vi "Lookup Message Channels.vi"(8 "error in (no error)":errorcluster, 10 "Message Channels in":T3 {"Status" format="%.0x"; "Triggers" format="%.0x"; "Periodic Enable" format="%.0x"}, 11 "Section Ref in":T2 format="%.0x") -> (0 "error out":errorcluster, 1 "Trigger Parameters":T1, 2 "Message Channels out":T3 {"Status" format="%.0x"; "Triggers" format="%.0x"; "Periodic Enable" format="%.0x"}, 3 "Section Ref out":T2 format="%.0x")   [LabVIEW 2015, in "Instrument Addon System Explorer.lvlib"]
uses:
  Instrument Addon System Explorer.lvlib
  Types/Message Channel Lookup Cluster.ctl
  <vilib>/NI Veristand/Custom Device API/Custom Device Item Ref.ctl
  Shared/Types/Trigger Parameters.ctl
  Shared/Types/FG Control.ctl
  <vilib>/NI Veristand/Custom Device Tools/Custom Device Utility Library/NI VeriStand - Search for Item by GUID.vi
  <vilib>/NI Veristand/Custom Device API/NI VeriStand - Set Item Property.vi
  <vilib>/NI Veristand/Custom Device API/Set Item Property (String).vi
  <vilib>/NI Veristand/Custom Device API/Set Item Property (Boolean).vi
  <vilib>/NI Veristand/Custom Device API/NI VeriStand - Get Item Property.vi
  <vilib>/NI Veristand/Custom Device API/Get Item Property (String).vi
  <vilib>/NI Veristand/Custom Device API/Get Item Property (Boolean).vi
  Shared/Constants.vi
  <vilib>/NI Veristand/Custom Device Tools/Custom Device Utility Library/Custom Device Utility Library.lvlib
  Shared/Instrument Addon Shared.lvlib
  <vilib>/NI VeriStand/Custom Device API/Custom Device API.lvlib
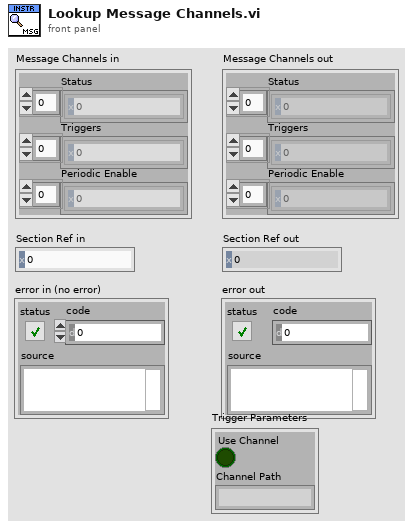
[diagram p1: front panel]
types:
  T1 = typedef "Instrument Addon Shared.lvlib/Trigger Parameters.ctl" = cluster{"Use Channel":bool, "Channel Path":string}
  T2 = typedef "Custom Device API.lvlib/Custom Device Item Ref.ctl" = u64
  T3 = typedef "Instrument Addon System Explorer.lvlib/Message Channel Lookup Cluster.ctl" = cluster{"Status":T2[], "Triggers":T2[], "Periodic Enable":T2[]}
  T4 = typedef "Instrument Addon Shared.lvlib/FG Control.ctl" = enum16{"Get", "Set"}
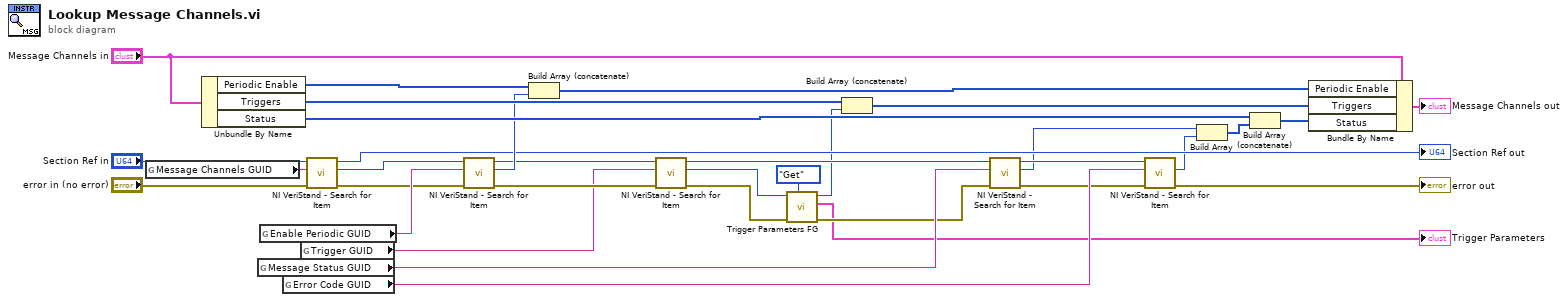
[diagram p0: block diagram]
diagram:
  n1 = global read "Constants.vi" "Message Channels GUID"() -> (w9:string)
  n2 = Unbundle By Name("Message Channels in") -> ("Periodic Enable"=w29:T2[], "Triggers"=w30:T2[], "Status"=w31:T2[])
  n3 = global read "Constants.vi" "Message Status GUID"() -> (w14:string)
  n4 = global read "Constants.vi" "Enable Periodic GUID"() -> (w27:string)
  n5 = global read "Constants.vi" "Error Code GUID"() -> (w13:string)
  n6 = global read "Constants.vi" "Trigger GUID"() -> (w15:string)
  n7 = call-poly <vilib>:"NI VeriStand - Search for Item.vi"("error in"="error in (no error)", "Item GUID"=w9, "Section Ref in"="Section Ref in") -> ("error out"=w25:errorcluster, "Item Ref"=w23:T2, "Section Ref out"=→"Section Ref out":T2)  [unwired: 5 in, 1 out]
  n8 = call-poly <vilib>:"NI VeriStand - Search for Item.vi"("error in"=w25, "Item GUID"=w27, "Section Ref in"=w23) -> ("error out"=w26:errorcluster, "Item Ref"=w28:T2, "Section Ref out"=w24:T2)  [unwired: 5 in, 1 out]
  n9 = Build Array (concatenate)(w29, w28) -> (w32:T2[])
  n10 = call-poly <vilib>:"NI VeriStand - Search for Item.vi"("error in"=w26, "Item GUID"=w15, "Section Ref in"=w24) -> ("error out"=w3:errorcluster, "Item Ref"=w6:T2, "Section Ref out"=w12:T2)  [unwired: 5 in, 1 out]
  n11 = call "Trigger Parameters FG.vi"("Action"=FG_Control."Get", "error in (no error)"=w3, "Item Ref in"=w6) -> ("error out"=w2:errorcluster, "Trigger Parameters"=→"Trigger Parameters":T1, "Item Ref out"=w5:T2)  [unwired: 6 in]
  n12 = Build Array (concatenate)(w30, w5) -> (w7:T2[])
  n13 = call-poly <vilib>:"NI VeriStand - Search for Item.vi"("error in"=w2, "Item GUID"=w14, "Section Ref in"=w12) -> ("error out"=w11:errorcluster, "Item Ref"=w16:T2, "Section Ref out"=w22:T2)  [unwired: 5 in, 1 out]
  n14 = call-poly <vilib>:"NI VeriStand - Search for Item.vi"("error in"=w11, "Item GUID"=w13, "Section Ref in"=w22) -> ("error out"=→"error out":errorcluster, "Item Ref"=w17:T2)  [unwired: 5 in, 2 out]
  n15 = Build Array(w16, w17) -> (w18:T2[])
  n16 = Build Array (concatenate)(w31, w18) -> (w8:T2[])
  n17 = Bundle By Name(cluster="Message Channels in", "Periodic Enable"=w32, "Triggers"=w7, "Status"=w8) -> (→"Message Channels out":T3)
